vi "UICtrls_Read_Name_(poly).vi"   [LabVIEW 2025]
uses:
  UI_Manager/UI_Manager.lvclass
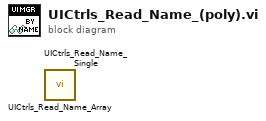
[diagram p0: block diagram]
diagram:
  n1 = call "UICtrls_Read_Name_Array.vi"() -> ()  [unwired: 8 in, 4 out]
  n2 = call "UICtrls_Read_Name_Single.vi"() -> ()  [unwired: 7 in, 5 out]
